vi "Format and Reverse.vi"(11 "String Input":string[](array[string])) -> (3 "Data Bytes":u8[](array[numeric]))   [LabVIEW 2014]
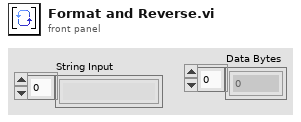
[diagram p1: front panel]
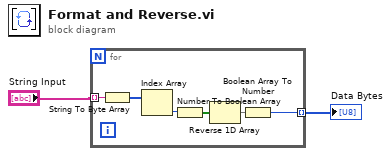
[diagram p0: block diagram]
diagram:
  n1 = for {
    tunnel: "String Input" -> [w7] mode=indexing
    tunnel: [w3] -> w1 mode=indexing
    n2 = String To Byte Array(string=w7) -> (unsigned byte array=w8:u8[])
    n3 = Index Array(array=w8) -> (element=w6:u8)  [unwired: 1 in]
    n4 = Number To Boolean Array(number=w6) -> (Boolean array=w5:bool[])
    n5 = Reverse 1D Array(array=w5) -> (reversed array=w4:bool[])
    n6 = Boolean Array To Number(Boolean array=w4) -> (number=w3:u32)
  }
  "Data Bytes" <- w1
